vi "Pack message frame.vi"(8 "error in":errorcluster, 9 "Size (bytes)":i32, 10 "Message Type":T1) -> (0 "error out":errorcluster, 2 "Message frame":u8[](array[numeric]) format="%b")   [LabVIEW 2020, in "wamplv.lvlib" / "RawSocket Handler.lvclass"]
uses:
  RawSocket Handler.lvclass
  Message Type.ctl
  RawSocket Handler.lvclass/RawSocket Handler.ctl
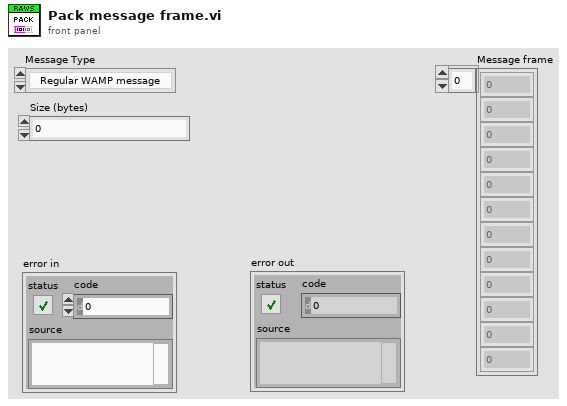
[diagram p1: front panel]
types:
  T1 = typedef "wamplv.lvlib/RawSocket Handler.lvclass/Message Type.ctl" = enum8{"Regular WAMP message", "PING", "PONG"}
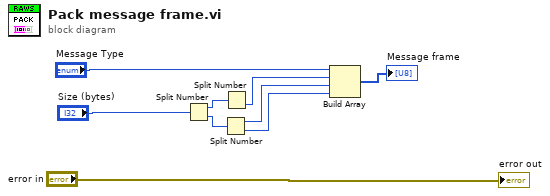
[diagram p0: block diagram]
diagram:
  n1 = Split Number(x="Size (bytes)") -> (hi(x)=w6:u16, lo(x)=w5:u16)
  n2 = Split Number(x=w5) -> (hi(x)=w3:u8, lo(x)=w2:u8)
  n3 = Split Number(x=w6) -> (lo(x)=w4:u8)  [unwired: 1 out]
  n4 = Build Array("Message Type", w4, w3, w2) -> (→"Message frame":u8[])
  "error out" <- "error in"
